vi "WaveformDataEventHandler Event Callback (DBL).vi"(4 "user event":refnum<user-event>, 5 "Event Data":cluster{"sender":refnum<k24>, "e":refnum<k24>}, 6 "Control Ref":refnum<k24>, 7 "Event Common Data":T1) -> ()   [LabVIEW 2020, in "NI_VS Waveform Streaming Interface.lvlib"]
uses:
  <vilib>/NI VeriStand/Execution/WaveformStreaming/NI_VS Waveform Streaming Interface.lvlib
  NationalInstruments.VeriStand.ClientAPI
  <vilib>/NI VeriStand/Execution/WaveformStreaming/Waveform Data Watcher Event Data (DBL).ctl
  <vilib>/NI VeriStand/Execution/WaveformStreaming/WaveformStreamSpecification.ctl
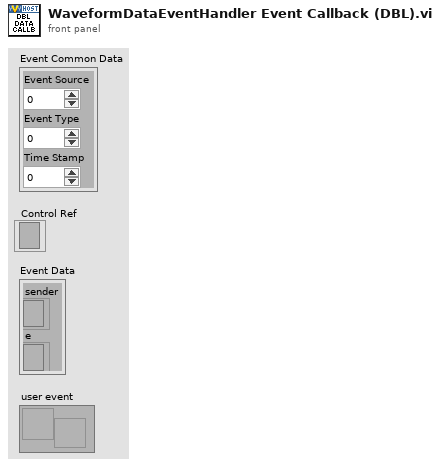
[diagram p1: front panel]
types:
  T1 = cluster{"Event Source":i32, "Event Type":u32, "Time Stamp":u32}
  T2 = typedef "NI_VS Waveform Streaming Interface.lvlib/Waveform Data Watcher Event Data (DBL).ctl" = cluster{"Data":dbl[], "dt":dbl, "offset from start (samples)":u64, "t0 at start":timestamp, "WaveformStreamSpecification":T3}
  T3 = typedef "NI_VS Waveform Streaming Interface.lvlib/WaveformStreamSpecification.ctl" = refnum<k24>
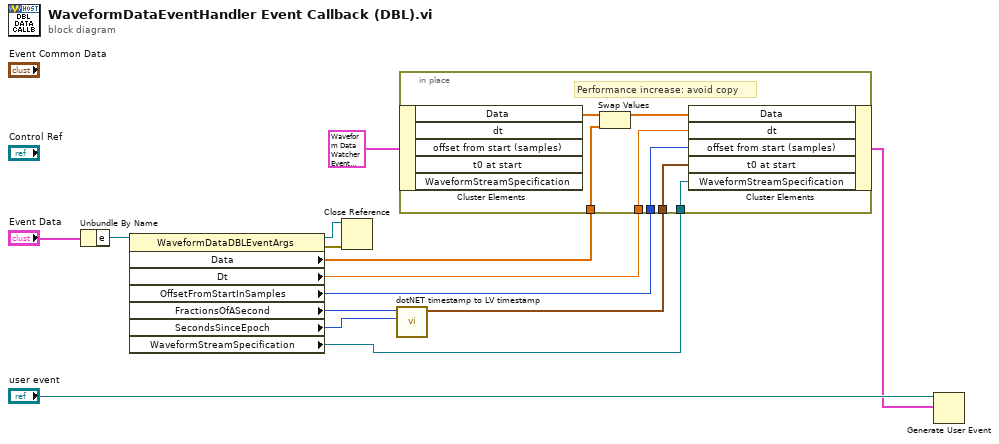
[diagram p0: block diagram]
diagram:
  n1 = Unbundle By Name("Event Data") -> ("e"=w12:refnum<k24>)
  n2 = property class="WaveformDataDBLEventArgs"(reference=w12) -> (reference out=w3:refnum<k24>, error out=w4:errorcluster, "Data"=w10:dbl[], "Dt"=w9:dbl, "OffsetFromStartInSamples"=w8:u64, "FractionsOfASecond"=w2:u64, "SecondsSinceEpoch"=w1:i64, "WaveformStreamSpecification"=w6:refnum<k24>)  [unwired: 1 in]
  n3 = Close Reference(reference=w3, error in (no error)=w4) -> ()  [unwired: 1 out]
  n4 = call <vilib>:"dotNET timestamp to LV timestamp.vi"("seconds since epoch"=w1, "positive fractions of a second"=w2) -> ("t0"=w7:timestamp)  [unwired: 9 in]
  n5 = in-place {
    in-place-border: w10 -> [w20]
    in-place-border: w9 -> [w18]
    in-place-border: w8 -> [w17]
    in-place-border: w7 -> [w16]
    in-place-border: w6 -> [w15]
    # "Performance increase: avoid copy"
    n6 = in-place-cluster #1(T2 {"Data"=[], "dt"=0.0, "offset from start (samples)"=0, "t0 at start"=timestamp(0 s since 1904-01-01), "WaveformStreamSpecification"=refnum} ("event data")) -> ("Data"=w21:dbl[])  [unwired: 4 out]
    n7 = Swap Values(12:w21, 14:w20) -> (1:w19:dbl[])  [unwired: 1 in, 1 out]
    n8 = in-place-cluster #1("Data"=w19, "dt"=w18, "offset from start (samples)"=w17, "t0 at start"=w16, "WaveformStreamSpecification"=w15) -> (w5:T2)
  }
  n9 = Generate User Event(user event="user event", event data cluster=w5) -> ()  [unwired: 2 in, 2 out]
